vi "Get Owning Custom Device.vi"(8 "error in":errorcluster, 11 "item ref in":T1 format="%.0x") -> (0 "error out":errorcluster, 2 "owning AIM ARINC-429 custom device":T1=18446744073709551615 format="%.0x", 3 "item ref out":T1 format="%.0x")   [LabVIEW 2024, in "AIM ARINC 429 Scripting.lvlib"]
uses:
  AIM ARINC 429 Scripting.lvlib
  <vilib>/NI VeriStand/Custom Device API/Custom Device Item Ref.ctl
  <vilib>/NI VeriStand/Custom Device Tools/Custom Device Utility Library/Search Direction.ctl
  Constants.vi
  <vilib>/NI VeriStand/Custom Device Tools/Custom Device Utility Library/NI VeriStand - Search for Item by GUID.vi
  <vilib>/NI VeriStand/Custom Device Tools/Custom Device Utility Library/Custom Device Utility Library.lvlib
  <vilib>/NI VeriStand/Custom Device API/Custom Device API.lvlib
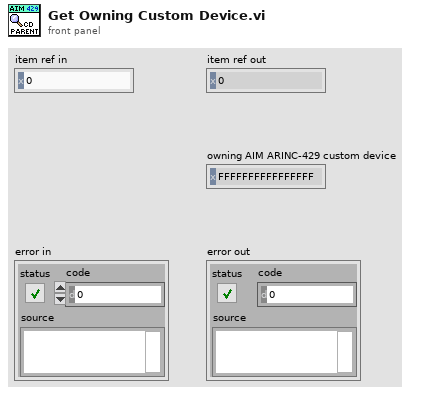
[diagram p1: front panel]
types:
  T1 = typedef "Custom Device API.lvlib/Custom Device Item Ref.ctl" = u64
  T2 = typedef "Custom Device Utility Library.lvlib/Search Direction.ctl" = enum16{"Down", "Up"}
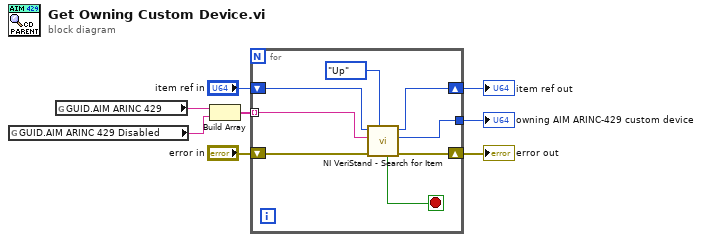
[diagram p0: block diagram]
diagram:
  n1 = global read "Constants.vi" "GUID.AIM ARINC 429 Disabled"() -> (w1:string)
  n2 = global read "Constants.vi" "GUID.AIM ARINC 429"() -> (w2:string)
  n3 = Build Array(w2, w1) -> (w3:string[])
  n4 = for {
    tunnel: [w10] -> w7
    tunnel: w3 -> [w12] mode=indexing
    shift-right: [w14] -> w5
    shift-left: "error in" -> [w15]
    shift-right: [w13] -> w4
    shift-left: "item ref in" -> [w16]
    stop <- w9 stop-if-true
    n5 = call-poly <vilib>:"NI VeriStand - Search for Item.vi"("Direction (Down)"=Search_Direction."Up", "error in"=w15, "Item GUID"=w12, "Section Ref in"=w16) -> ("error out"=w14:errorcluster, "Item Ref"=w10:T1, "Section Ref out"=w13:T1, "Found"=w9:bool)  [unwired: 4 in]
  }
  "owning AIM ARINC-429 custom device" <- w7
  "error out" <- w5
  "item ref out" <- w4
